vi "Get Named Range Values (Boolean).vi"(8 "error in":errorcluster, 9 "Sheet Name":string, 10 "Named Range Identifier":string, 11 "SpreadsheetDoc in":refnum<k24>) -> (0 "error out":errorcluster, 2 "Cells":bool[][](array[boolean]), 3 "SpreadsheetDoc out":refnum<k24>)   [LabVIEW 2019, in "Open Xml.lvlib"]
uses:
  Open Xml.lvlib
  D:/git/Open-Xml-LabVIEW/Source/DocumentFormat.OpenXml.dll
  DocumentFormat.OpenXml.dll
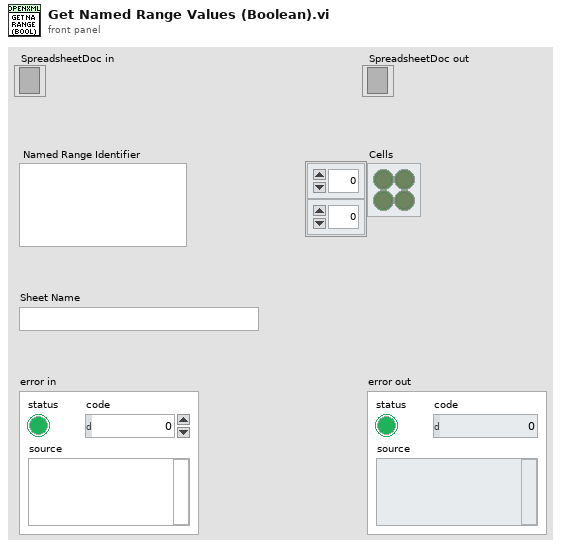
[diagram p1: front panel]
types:
  T1 = typedef "Open Xml.lvlib/Cell DataType.ctl" = enum16{"Void", "Boolean", "Number", "Error", "SharedString", "String", "InlineString", "Date"}
  T2 = cluster{"Number":dbl, "String":string, "Boolean":bool, "Time Stamp":timestamp, "Error":errorcluster}[][]
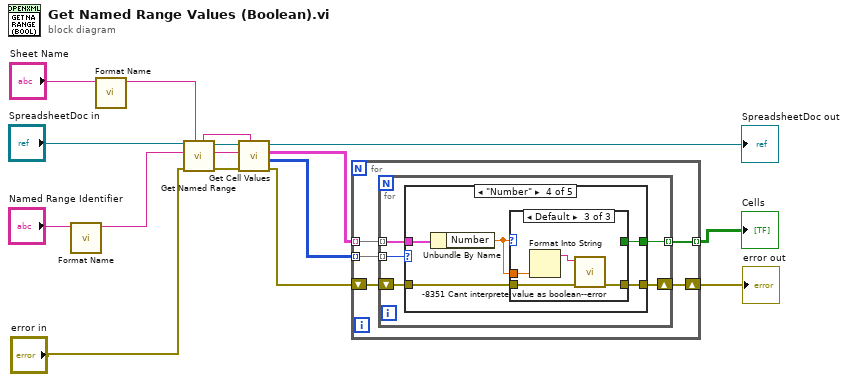
[diagram p0: block diagram]
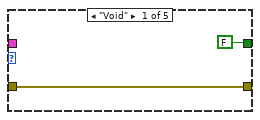
[diagram p2: hidden frame]
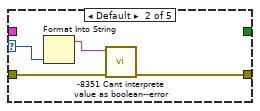
[diagram p3: hidden frame]
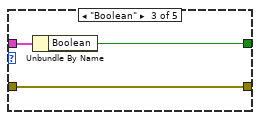
[diagram p4: hidden frame]
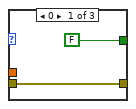
[diagram p5: hidden frame]
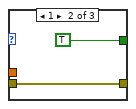
[diagram p6: hidden frame]
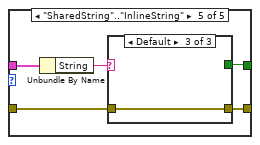
[diagram p7: hidden frame]
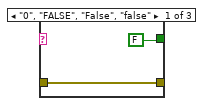
[diagram p8: hidden frame]
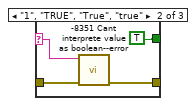
[diagram p9: hidden frame]
diagram:
  n1 = call "Format Name.vi"("Sheet Name"="Named Range Identifier") -> ("Formatted Sheet Name"=w2:string)  [unwired: 10 in]
  n2 = call "Format Name.vi"("Sheet Name"="Sheet Name") -> ("Formatted Sheet Name"=w1:string)  [unwired: 10 in]
  n3 = call "Get Named Range.vi"("Sheet Name"=w1, "error in"="error in", "Range Identifier"=w2, "SpreadsheetDoc in"="SpreadsheetDoc in") -> ("error out"=w13:errorcluster, "Range"=w10:string, "SpreadsheetDoc out"=w12:refnum<k24>, "Sheet Name"=w11:string)  [unwired: 4 in]
  n4 = call "Get Cell Values.vi"("Sheet Name"=w11, "error in"=w13, "Cell Addresses"=w10, "SpreadsheetDoc in"=w12) -> ("error out"=w5:errorcluster, "Types"=w7:T1[][], "Cell Values"=w9:T2, "SpreadsheetDoc out"=→"SpreadsheetDoc out":refnum<k24>)  [unwired: 4 in]
  n5 = for {
    tunnel: w9 -> [w21] mode=indexing
    tunnel: w7 -> [w20] mode=indexing
    tunnel: [w19] -> w3 mode=indexing
    shift-right: [w17] -> w4
    shift-left: w5 -> [w18]
    n6 = for {
      tunnel: w21 -> [w25] mode=indexing
      tunnel: w20 -> [w26] mode=indexing
      tunnel: [w22] -> w19 mode=indexing
      shift-right: [w23] -> w17
      shift-left: w18 -> [w24]
      n7 = case shown="\"Number\"" w26 {
        selector: w26 -> [_ w30 _ _ _]
        tunnel: w25 -> [_ _ w35 w40 w53]
        tunnel: [FALSE _ w34 w39 w51] -> w22
        tunnel: w24 -> [w27 w32 w33 w38 w50]
        tunnel: [w27 w31 w33 w37 w49] -> w23
        frame "Void" {
        }
        frame Default {
          n8 = Format Into String(w30) -> (resulting string=w29:string)  [unwired: 3 in, 1 out]
          n9 = call "-8351 Cant interprete value as boolean--error.vi"("error in"=w32, "Argument"=w29) -> ("error out"=w31:errorcluster)  [unwired: 8 in, 1 out]
        }
        frame "Boolean" {
          n10 = Unbundle By Name(w35) -> ("Boolean"=w34:bool)
        }
        frame "Number" {
          n11 = Unbundle By Name(w40) -> ("Number"=w36:dbl)
          n12 = case shown="Default" w36 {
            tunnel: [FALSE TRUE _] -> w39
            tunnel: w38 -> [w41 w43 w47]
            tunnel: [w41 w43 w48] -> w37
            tunnel: w36 -> [_ _ w46]
            frame 0 {
            }
            frame 1 {
            }
            frame Default {
              n13 = Format Into String(w46) -> (resulting string=w45:string)  [unwired: 3 in, 1 out]
              n14 = call "-8351 Cant interprete value as boolean--error.vi"("error in"=w47, "Argument"=w45) -> ("error out"=w48:errorcluster)  [unwired: 8 in, 1 out]
            }
          }
        }
        frame "SharedString".."InlineString" {
          n15 = Unbundle By Name(w53) -> ("String"=w52:string)
          n16 = case shown="Default" w52 {
            selector: w52 -> [_ w56 _]
            tunnel: [FALSE TRUE _] -> w51
            tunnel: w50 -> [w54 w58 w60]
            tunnel: [w54 w57 w60] -> w49
            frame "0", "FALSE", "False", "false" {
            }
            frame "1", "TRUE", "True", "true" {
              n17 = call "-8351 Cant interprete value as boolean--error.vi"("error in"=w58, "Argument"=w56) -> ("error out"=w57:errorcluster)  [unwired: 8 in, 1 out]
            }
            frame Default {
            }
          }
        }
      }
    }
  }
  "Cells" <- w3
  "error out" <- w4
